vi "WriteMbDat.vi"(0 "ModbusSp in":refnum<class "ModbusSp.lvclass">, 5 "Data Write":T1, 11 "error in (no error)":errorcluster) -> (4 "ModbusSp out":refnum<class "ModbusSp.lvclass">, 6 "registers to write":u16[](array[numeric]), 15 "error out":errorcluster)   [LabVIEW 2019, in "ModbusSp.lvclass"]
uses:
  ModbusSp.lvclass
  WriteData.ctl
  ModbusSp.lvclass/ModbusSp.ctl
  Modbus Data Type Conversation/SGL Array to U16 Array.vi
  Modbus Data Type Conversation/SGL to U16.vi
  <vilib>/NI/Modbus Library/API/Slave/Modbus Slave.lvclass
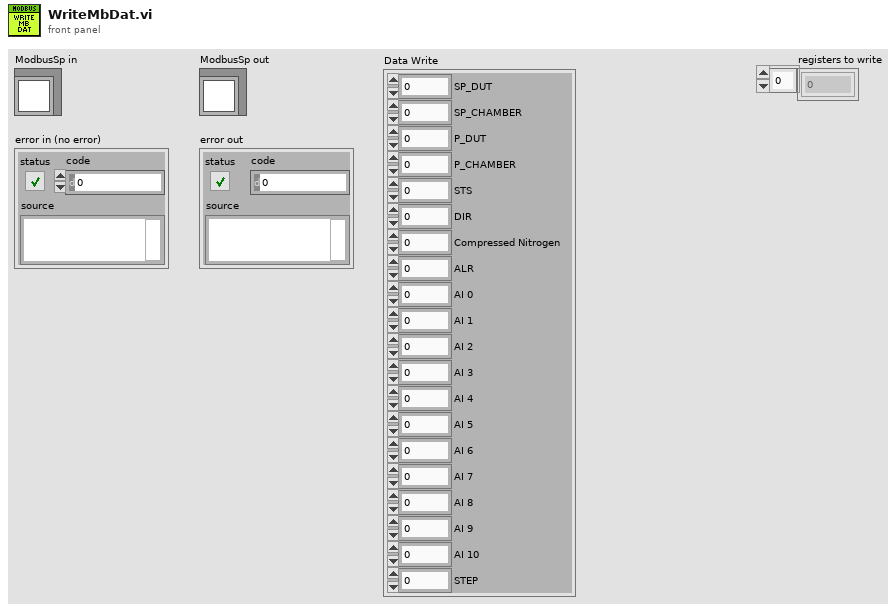
[diagram p1: front panel]
types:
  T1 = typedef "ModbusSp.lvclass/WriteData.ctl" = cluster{"SP_DUT":sgl, "SP_CHAMBER":sgl, "P_DUT":sgl, "P_CHAMBER":sgl, "STS":u16, "DIR":u16, "Compressed Nitrogen":u16, "ALR":u16, "AI 0":sgl, "AI 1":sgl, "AI 2":sgl, "AI 3":sgl, "AI 4":sgl, "AI 5":sgl, "AI 6":sgl, "AI 7":sgl, "AI 8":sgl, "AI 9":sgl, "AI 10":sgl, "STEP":u16}
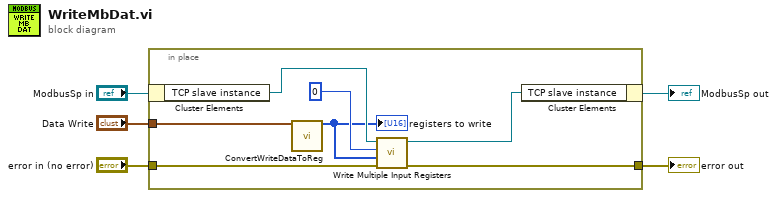
[diagram p0: block diagram]
diagram:
  n1 = in-place {
    in-place-border: [w10] -> w5
    in-place-border: "error in (no error)" -> [w8]
    in-place-border: "Data Write" -> [w6]
    n2 = in-place-cluster #1("ModbusSp in") -> ("TCP slave instance"=w12:refnum<class "Modbus Slave.lvclass">)
    n3 = call "ConvertWriteDataToReg.vi"("SharedData Write"=w6) -> ("registers to write"=w7:u16[])  [unwired: 14 in]
    "registers to write" <- w7
    n4 = call-dynamic "Write Multiple Input Registers.vi"("error in"=w8, "input registers to write"=w7, "starting address"=u16 0, "Modbus slave in"=w12) -> ("error out"=w10:errorcluster, "Modbus slave out"=w11:refnum<class "Modbus Slave.lvclass">)  [unwired: 6 in]
    n5 = in-place-cluster #1("TCP slave instance"=w11) -> (→"ModbusSp out":refnum<class "ModbusSp.lvclass">)
  }
  "error out" <- w5
